vi "Configure Trigger.vi"(8 "error in (no error)":errorcluster, 10 "Trigger Source (0: None)":u16(ring) items=["None", "Star Trigger"], 11 "VISA resource name":refnum<visa-resource-name>) -> (0 "error out":errorcluster, 3 "VISA resource name out":refnum<visa-resource-name>)   [LabVIEW 2018, in "Agilent U2722.lvlib"]
doc: "Configures the trigger source."
uses:
  <instrlib>/Agilent U2722/Agilent U2722.lvlib
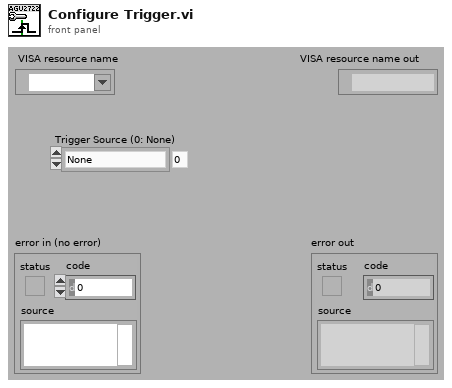
[diagram p1: front panel]
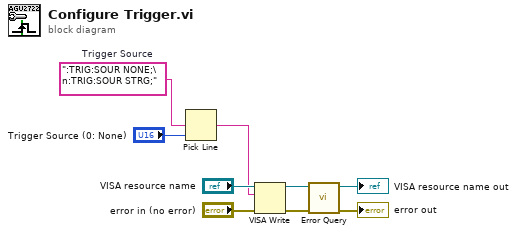
[diagram p0: block diagram]
diagram:
  w6 = ":TRIG:SOUR NONE;\n:TRIG:SOUR STRG;"  # Trigger Source
  n1 = Pick Line(multi-line string=w6, line index="Trigger Source (0: None)") -> (output string=w1:string)  [unwired: 1 in]
  n2 = VISA Write(VISA resource name="VISA resource name", write buffer=w1, error in (no error)="error in (no error)") -> (VISA resource name out=w3:refnum<visa-resource-name>, error out=w2:errorcluster)  [unwired: 1 out]
  n3 = call <instrlib>:"Error Query.vi"("error in (no error)"=w2, "VISA resource name"=w3) -> ("error out"=→"error out":errorcluster, "VISA resource name out"=→"VISA resource name out":refnum<visa-resource-name>)  [unwired: 6 in, 2 out]
